vi "Get VI Reference.vi"(8 "error in (no error)":errorcluster, 11 "SMO UI":refnum<class "SMO.UI.Embedded.lvclass">) -> (0 "error out":errorcluster, 2 "VI Reference":refnum<vi>, 3 "SMO UI out":refnum<class "SMO.UI.Embedded.lvclass">)   [LabVIEW 2020, in "SMO.UI.Embedded.lvclass"]
doc: "JKI State Machine Objects (SMO) 1.3.0.56\nJKI - JKI\nCopyright (c) 2017, JKI"
uses:
  SMO.UI.Embedded.lvclass
  <vilib>/JKI/JKI SMO/SMO.UI/SMO.UI.lvclass
panel:
  # "For instructions on how to use the JKI State Machine Objects, examples and video tutorials, visit:\nhttp://jki.net/state-machine-objects/\n\nJKI State Machine Objects™\nhttp://jki.net/state-machine-objects/\nCopyright (C) 2005-2015, JKI <info@jki.net>\nALL RIGHTS RESERVED"
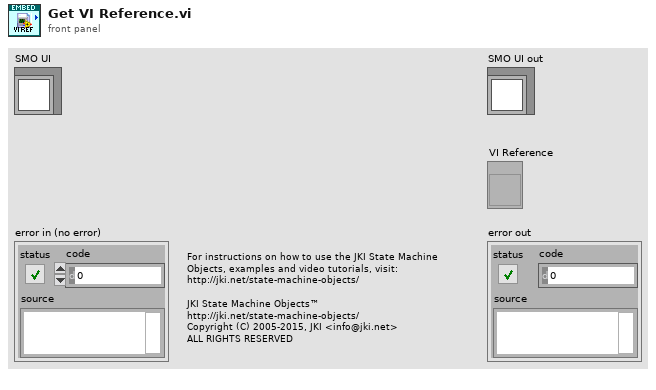
[diagram p1: front panel]
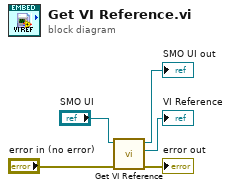
[diagram p0: block diagram]
diagram:
  n1 = call-parent "Get VI Reference.vi"("error in (no error)"="error in (no error)", "SMO UI"="SMO UI") -> ("error out"=→"error out":errorcluster, "VI Reference"=→"VI Reference":refnum<vi>, "SMO UI out"=→"SMO UI out":refnum<class "SMO.UI.Embedded.lvclass">)  [unwired: 7 in]
